vi "8bit sync-AVI cleanup.vi"(8 "error in (no error)":errorcluster, 11 "Output AVI ref":T1) -> ()   [LabVIEW 2020]
uses:
  <vilib>/vision/Avi.llb/IMAQ AVI2 Refnum.ctl
  Globals/gl_8-bit montage window ctrl refs.vi
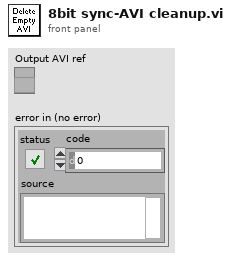
[diagram p1: front panel]
types:
  T1 = typedef "IMAQ AVI2 Refnum.ctl" = refnum<k20>
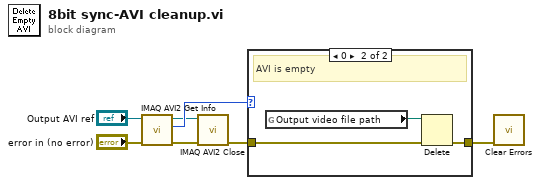
[diagram p0: block diagram]
diagram:
  n1 = call "IMAQ AVI2 Get Info"("error in (no error)"="error in (no error)", "AVI Refnum"="Output AVI ref") -> ("error out"=w4:errorcluster, "Number of Frames"=w5:u32, "AVI Refnum (duplicate)"=w2:T1)  [unwired: 5 in, 2 out]
  n2 = call "IMAQ AVI2 Close"("error in (no error)"=w4, "AVI Refnum"=w2) -> ("error out"=w3:errorcluster)  [unwired: 9 in]
  n3 = case shown="0" w5 {
    tunnel: w3 -> [w8 w11]
    tunnel: [w8 w10] -> w1
    frame Default {
      # "AVI is not empty"
    }
    frame 0 {
      # "AVI is empty"
      n4 = global read "gl_8-bit montage window ctrl refs.vi" "Output video file path"() -> (w9:path)
      n5 = Delete(path (use dialog)=w9, error in=w11) -> (error out=w10:errorcluster)  [unwired: 3 in, 2 out]
    }
  }
  n6 = call <vilib>:"Clear Errors.vi"("error in (no error)"=w1) -> ()  [unwired: 5 in, 2 out]
